vi "Action_2.vi"(1 "Time Since Latch":u32, 2 "Instruction String":string) -> (0 "Advance Trigger":bool)   [LabVIEW 2018]
uses:
  Global_Commands.vi
  Global_Sensors.vi
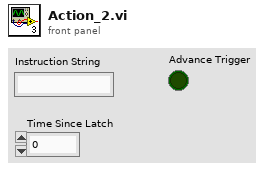
[diagram p1: front panel]
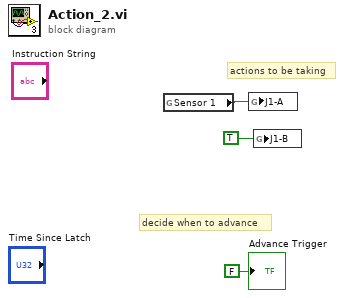
[diagram p0: block diagram]
diagram:
  # "actions to be taking"
  # "decide when to advance"
  n1 = global read "Global_Sensors.vi" "Sensor 1"() -> (w1:bool)
  n2 = global write "Global_Commands.vi" "J1-A"(w1) -> ()
  n3 = global write "Global_Commands.vi" "J1-B"(TRUE) -> ()
  "Advance Trigger" <- FALSE ("Advance Trigger")
